vi "Generate snapshot or ref folder path.vi"(8 "error in (no error)":errorcluster) -> (0 "error out":errorcluster, 3 "Snapshot folder path":path)   [LabVIEW 2017]
uses:
  Global Variables/General Globals.vi
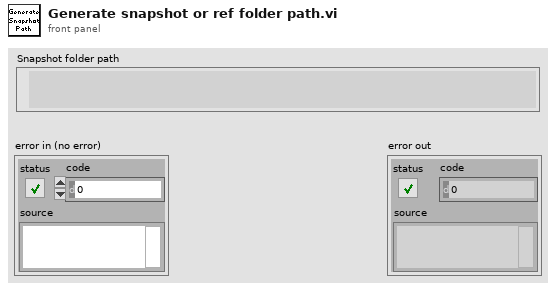
[diagram p1: front panel]
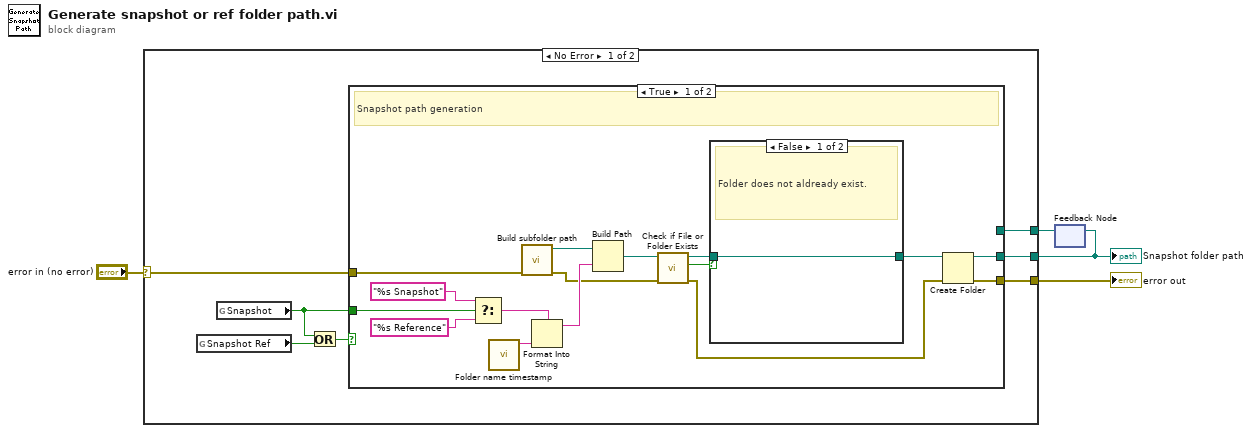
[diagram p0: block diagram]
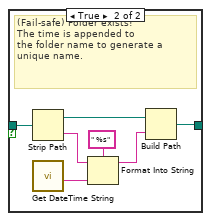
[diagram p2: hidden frame]
diagram:
  n1 = feedback #1() -> (w1:path)  [unwired: 1 in]
  n2 = case shown="No Error" "error in (no error)" {
    selector: "error in (no error)" -> [w5 w37]
    tunnel: [w11 w37] -> w4
    tunnel: [w10 w38] -> w2
    tunnel: w1 -> [w9 w38]
    frame No Error {
      n3 = global read "General Globals.vi" "Snapshot Ref"() -> (w8:bool)
      n4 = global read "General Globals.vi" "Snapshot"() -> (w6:bool)
      n5 = Or(x=w6, y=w8) -> (x .or. y?=w7:bool)
      n6 = case shown="True" w7 {
        tunnel: [w15 w36] -> w10
        tunnel: [w17 _] -> w11
        tunnel: w9 -> [_ w36]
        tunnel: w6 -> [w22 _]
        tunnel: w5 -> [w13 _]
        frame True {
          # "Snapshot path generation"
          n7 = Select(t="%s Snapshot" ("name or relative path"), s=w22, f="%s Reference" ("name or relative path")) -> (s? t:f=w21:string)
          n8 = call "Folder name timestamp.vi"() -> ("date/time string"=w19:string)  [unwired: 11 in]
          n9 = call "Build subfolder path.vi"("error in (no error)"=w13) -> ("error out"=w12:errorcluster, "Daily folder or sub-folder path"=w18:path)  [unwired: 9 in]
          n10 = Format Into String(format string=w21, w19) -> (resulting string=w20:string)  [unwired: 2 in, 1 out]
          n11 = Build Path(base path=w18, name or relative path=w20) -> (appended path=w25:path)
          n12 = call <vilib>:"Check if File or Folder Exists.vi"("error in (no error)"=w12, "path"=w25) -> ("error out"=w16:errorcluster, "file or folder exists?"=w26:bool, "dup path"=w27:path)  [unwired: 7 in]
          n13 = case shown="False" w26 {
            tunnel: [w28 w30] -> w14
            tunnel: w27 -> [w28 w34]
            frame False {
              # "Folder does not aldready exist."
            }
            frame True {
              # "(Fail-safe) Folder exists!\nThe time is appended to\nthe folder name to generate a unique name."
              n14 = Strip Path(path=w34) -> (stripped path=w35:path, name=w29:string)
              n15 = call <userlib>:"Get DateTime String.vi"() -> ("Time string"=w33:string)  [unwired: 10 in, 1 out]
              n16 = Format Into String(format string=" %s", initial string=w29, w33) -> (resulting string=w31:string)  [unwired: 1 in, 1 out]
              n17 = Build Path(base path=w35, name or relative path=w31) -> (appended path=w30:path)
            }
          }
          n18 = Create Folder(path (use dialog)=w14, error in=w16) -> (created path=w15:path, error out=w17:errorcluster)  [unwired: 1 in, 1 out]
        }
        frame False {
        }
      }
    }
    frame Error {
    }
  }
  "Snapshot folder path" <- w2
  "error out" <- w4
  n19 = feedback-in #1(w2) -> ()
